vi "Find Straight Edge.vi"(6 "Analysis_Setting IN":T2={"PreProcess"=enum."*Algorithm*", "Parameter"=""}, 8 "error in (no error)":errorcluster, 9 "ProjectName":string, 10 "ROI List IN":refnum<vi>, 11 "Vision_Image":T12(plugin-control)) -> (0 "error out":errorcluster, 1 "Cancel?":bool, 3 "Analysis_Setting":T2={"PreProcess"=enum."*Algorithm*", "Parameter"=""})   [LabVIEW 2019]
uses:
  <vilib>/userdefined/High Color/IMAQdx.ctl
  <vilib>/vision/NI_Vision_Development_Module.lvlib
  Controls/Analysis_Type.ctl
  Controls/Analysis_Setting.ctl
  Controls/_UI Command Cluster/Find Straight Edge_UI Command Cluster.ctl
  Controls/Find Straight Edge/Analysis_Find Straight Edge_Parameter.ctl
  <vilib>/vision/Measure.llb/Straight Edge Process.ctl
  <vilib>/vision/Measure.llb/Straight Edge Options.ctl
  <vilib>/vision/Measure.llb/Edge Polarity.ctl
  <vilib>/vision/Measure.llb/Edge Options.ctl
  Controls/V_Analysis_Type.ctl
  Ctrl/VisionProcessName.ctl
panel:
  in  "Number of Matches Requested":i32=1 min=1 max=9999
  in  "Snap?":bool
  out "Edge Info Size":i32
  in  "ROI":T1
  out "Numeric":i32
  in  "Done":bool
  in  "Straight Edge_UI Command":T4(ring)
  in  "Cancel":bool
  in  "Straight EdgeTab":T5(tab)
  in  "Options":T8={"Search Direction"=0, "Edge Options"={"Edge Polarity"=0, "Kernel Size"=3, "Width"=3, "Minimum Edge Strength"=10.0, "Interpolation Type"=enum."Bilinear Fixed", "Data Processing Method"=enum."Average"}, "Show Search Area"=FALSE, "Show Search Lines"=FALSE, "Show Edges Found"=FALSE, "Show Result"=TRUE, "Search Area Color"=65280, "Search Lines Color"=255, "Edge Locations Color"=16776960, "Result Color"=16711680, "Overlay Group Name"=""} {"Edge Options"."Edge Polarity" items=["All Edges", "Rising Edges", "Falling Edges"]; "Edge Options"."Minimum Edge Strength" format="%.2f"; "Edge Options"."Width" step=2; "Edge Options"."Kernel Size" min=3 step=2; "Search Direction" items=["Left to Right", "Right to Left", "Top to Bottom", "Bottom to Top"]}
  in  "Line Fit Options":T9={"Number of Lines"=1, "Type"=enum."First Edge Rake", "Min. Score"=10.0, "Max. Score"=1000.0, "Orientation"=0.0, "Angle Range"=45.0, "Angle Tolerance"=1.0, "Step Size"=7, "Min. SNR (db)"=0.0, "Min. Points (%)"=25.0, "Hough Iterations"=5} {"Min. Points (%)" min=0.0 max=100.0; "Min. SNR (db)" min=0.0; "Max. Score" min=0.0 max=1024.0; "Min. Score" min=0.0 max=1024.0 step=1.0}
  out "Straight Edges":T11(array[cluster]) {"Point2 (Real-World)"."Y" format="%.2f"; "Point2 (Real-World)"."X" format="%.2f"; "Point1 (Real-World)"."Y" format="%.2f"; "Point1 (Real-World)"."X" format="%.2f"; "Point2 (Pixels)"."Y" format="%.2f"; "Point2 (Pixels)"."X" format="%.2f"; "Point1 (Pixels)"."Y" format="%.2f"; "Point1 (Pixels)"."X" format="%.2f"}
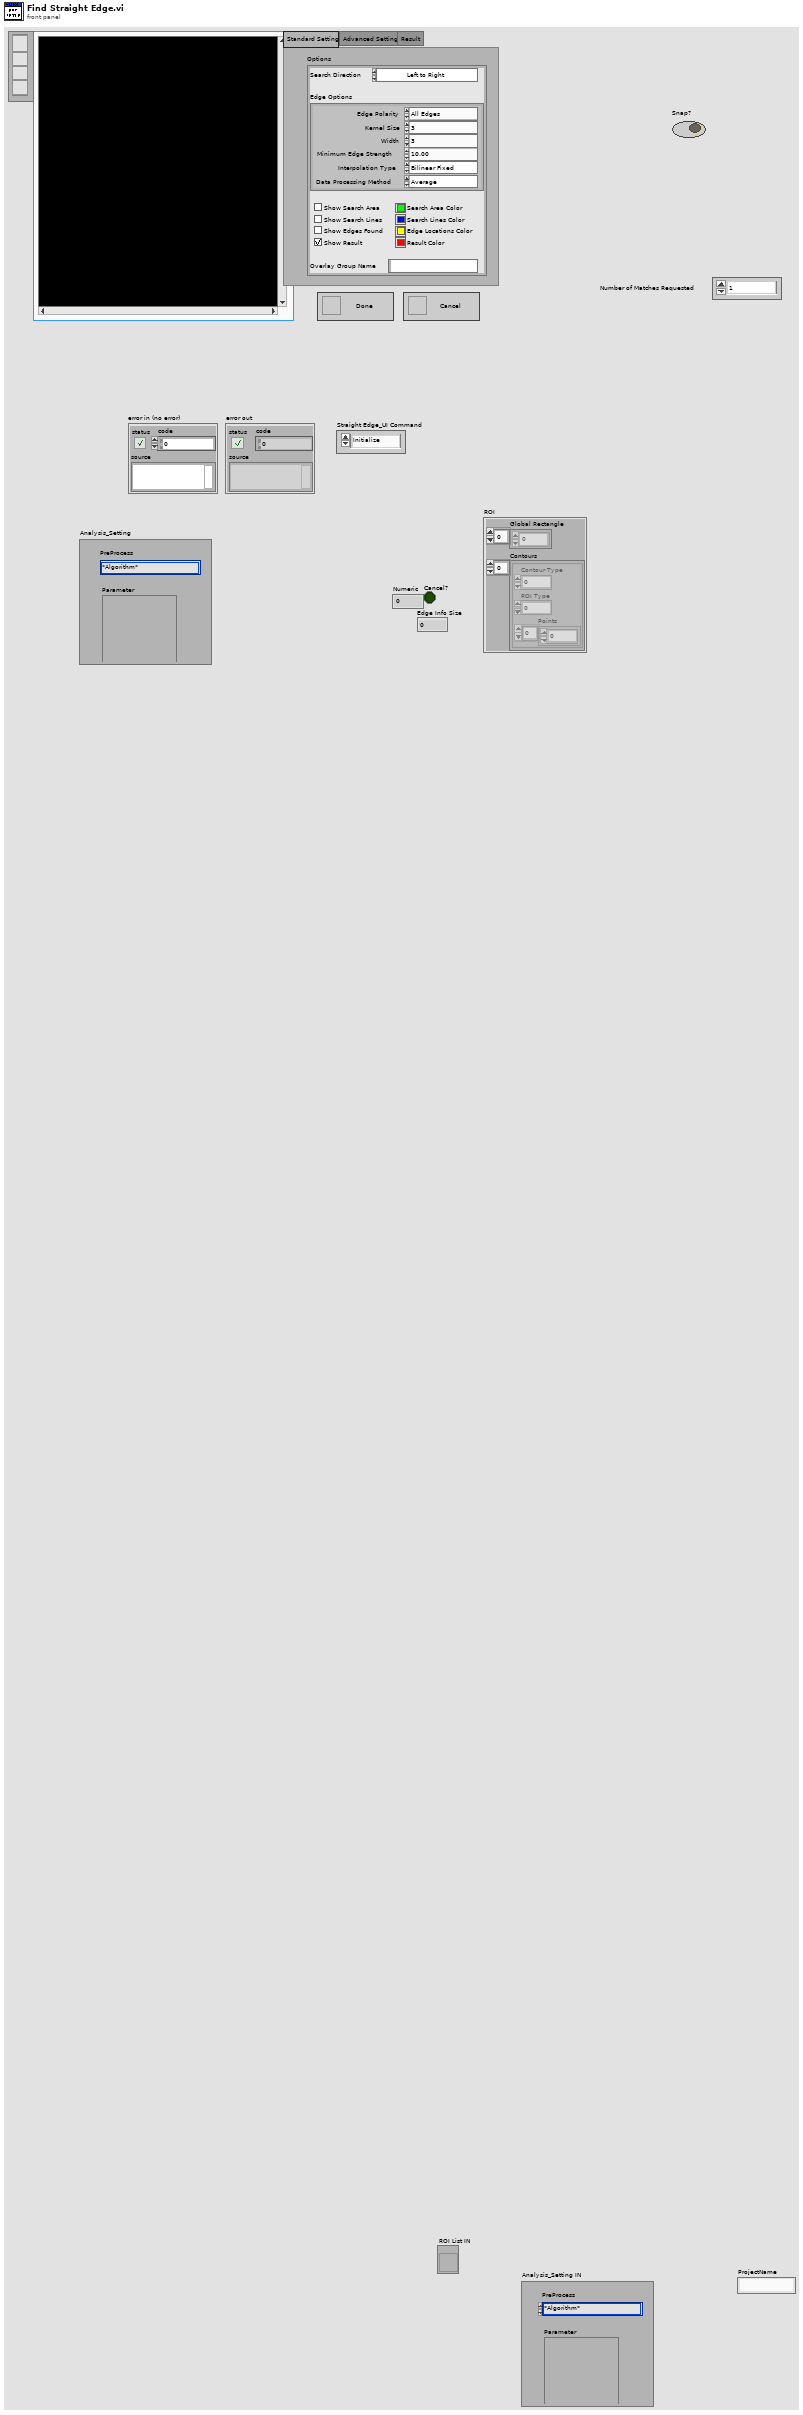
[diagram p1: front panel]
types:
  T1 = cluster{"Global Rectangle":i32[], "Contours":cluster{"Contour Type":u32, "ROI Type":u32, "Points":i32[]}[]}
  T2 = typedef "Analysis_Setting.ctl" = cluster{"PreProcess":T3, "Parameter":string}
  T3 = typedef "VisionProcessName.ctl" = enum16{"*CamParameter*", "CamAttributes", "*Preprocess*", "CG_Brightness", "C_Plane Extraction", "C_Threshold", "G_Lookup Table", "G_Threshold", "B_Image Inversion", "*Algorithm*", "CG_Histogram", "C_Color Matching", "C_Color Pattern Matching", "G_PatternMatch", "CG_Find Straight Edge", "CG_Adv. Find Straight Edge", "CG_Find Circular Edge", "G_Max Clamp", "G_Clamp (Rake)", "G_Pattern Matching"}
  T4 = enum16{"Initialize", "Done", "Run Algorithm", "Cancel"}
  T5 = enum32{"Standard Setting", "Advanced Setting", "Result"}
  T6 = typedef "Edge Options.ctl" = cluster{"Edge Polarity":T7, "Kernel Size":u32, "Width":u32, "Minimum Edge Strength":sgl, "Interpolation Type":enum32{"Zero Order", "Bilinear", "Quadratic", "Cubic", "Bilinear Fixed"}, "Data Processing Method":enum32{"Average", "Median"}}
  T7 = typedef "Edge Polarity.ctl" = u32
  T8 = cluster{"Search Direction":u32, "Edge Options":T6, "Show Search Area":bool, "Show Search Lines":bool, "Show Edges Found":bool, "Show Result":bool, "Search Area Color":u32, "Search Lines Color":u32, "Edge Locations Color":u32, "Result Color":u32, "Overlay Group Name":string}
  T9 = typedef "Straight Edge Options.ctl" = cluster{"Number of Lines":i32, "Type":T10, "Min. Score":dbl, "Max. Score":dbl, "Orientation":dbl, "Angle Range":dbl, "Angle Tolerance":dbl, "Step Size":u32, "Min. SNR (db)":dbl, "Min. Points (%)":dbl, "Hough Iterations":i32}
  T10 = typedef "Straight Edge Process.ctl" = enum32{"First Edge Rake", "Best Edge Rake", "Hough Edge Rake", "First Edge Projection", "Best Edge Projection"}
  T11 = cluster{"Point1 (Pixels)":cluster{"X":sgl, "Y":sgl}, "Point2 (Pixels)":cluster{"X":sgl, "Y":sgl}, "Point1 (Real-World)":cluster{"X":sgl, "Y":sgl}, "Point2 (Real-World)":cluster{"X":sgl, "Y":sgl}, "Angle (Pixel)":dbl, "Angle (Real-World)":dbl, "Score":dbl, "Straightness":dbl, "Average SNR (db)":dbl, "Calibration Valid":bool}[]
  T12 = typedef "IMAQ Image.ctl" = refnum<image>
  T13 = typedef "Find Straight Edge_UI Command Cluster.ctl" = cluster{"Find Straight Edge_UI Command":enum16{"Initialize", "Done", "Run Algorithm", "Cancel"}, "Snap Simulation Mouse Down":bool, "ROI Descriptor":cluster{"Global Rectangle":i32[], "Contours":cluster{"Contour Type":u32, "ROI Type":u32, "Points":i32[]}[]}, "Number of Matches Requested":i32, "Options":cluster{"Search Direction":u32, "Edge Options":T6, "Show Search Area":bool, "Show Search Lines":bool, "Show Edges Found":bool, "Show Result":bool, "Search Area Color":u32, "Search Lines Color":u32, "Edge Locations Color":u32, "Result Color":u32, "Overlay Group Name":string}, "Line Fit Options":T9}
  T14 = typedef "IMAQ Line" = cluster{"Start X":i32, "Start Y":i32, "End X":i32, "End Y":i32}
  T15 = typedef "IMAQdx.ctl" = refnum<k21>
  T16 = cluster{"Contour Type":u32, "ROI Type":u32, "Points":i32[]}
  T17 = typedef "Image Type" = u32
  T18 = typedef "Analysis_Find Straight Edge_Parameter.ctl" = cluster{"ROI Descriptor":cluster{"Global Rectangle":i32[], "Contours":cluster{"Contour Type":u32, "ROI Type":u32, "Points":i32[]}[]}, "Number of Matches Requested":i32, "Edge Info Size":i32, "Options":cluster{"Search Direction":u32, "Edge Options":T6, "Show Search Area":bool, "Show Search Lines":bool, "Show Edges Found":bool, "Show Result":bool, "Search Area Color":u32, "Search Lines Color":u32, "Edge Locations Color":u32, "Result Color":u32, "Overlay Group Name":string}, "Line Fit Options":T9}
  T19 = typedef "Analysis_Type.ctl" = u16
  T20 = typedef "Analysis_Setting.ctl" = cluster{"PreProcess":T21, "Parameter":string}
  T21 = typedef "V_Analysis_Type.ctl" = enum16{"None", "C_Color Pattern Matching", "G_PatternMatching", "G_ShapeDectect", "G_GeometricMatch", "B_Area Check"}
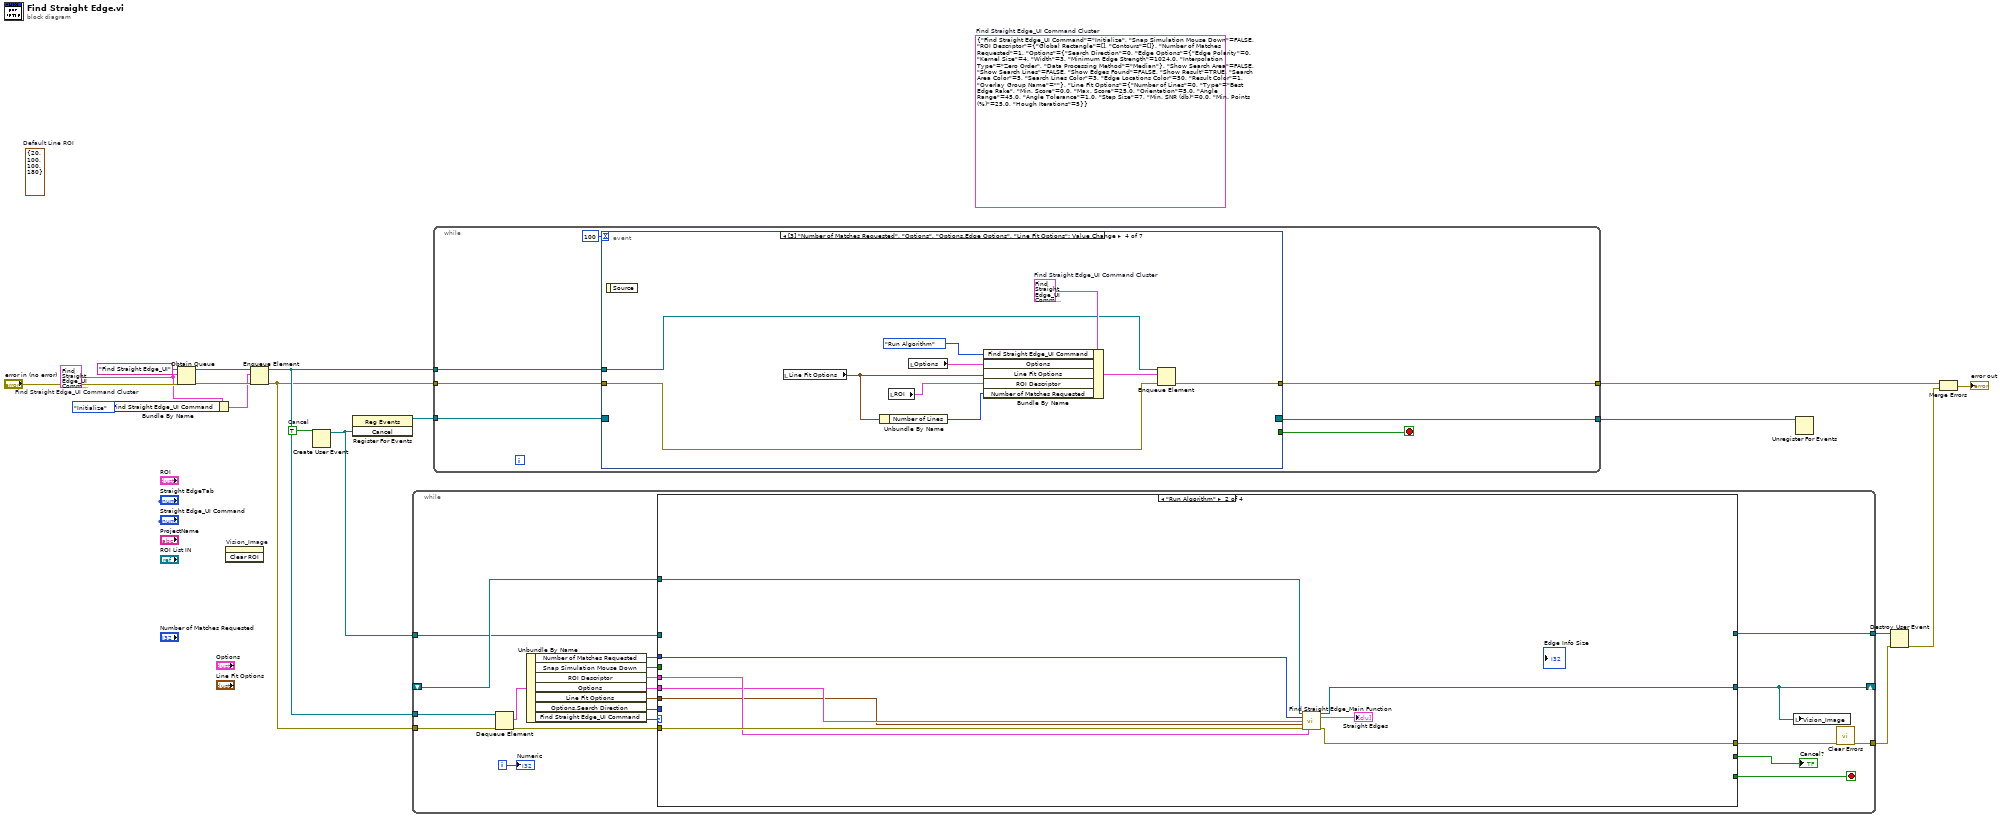
[diagram p0: block diagram]
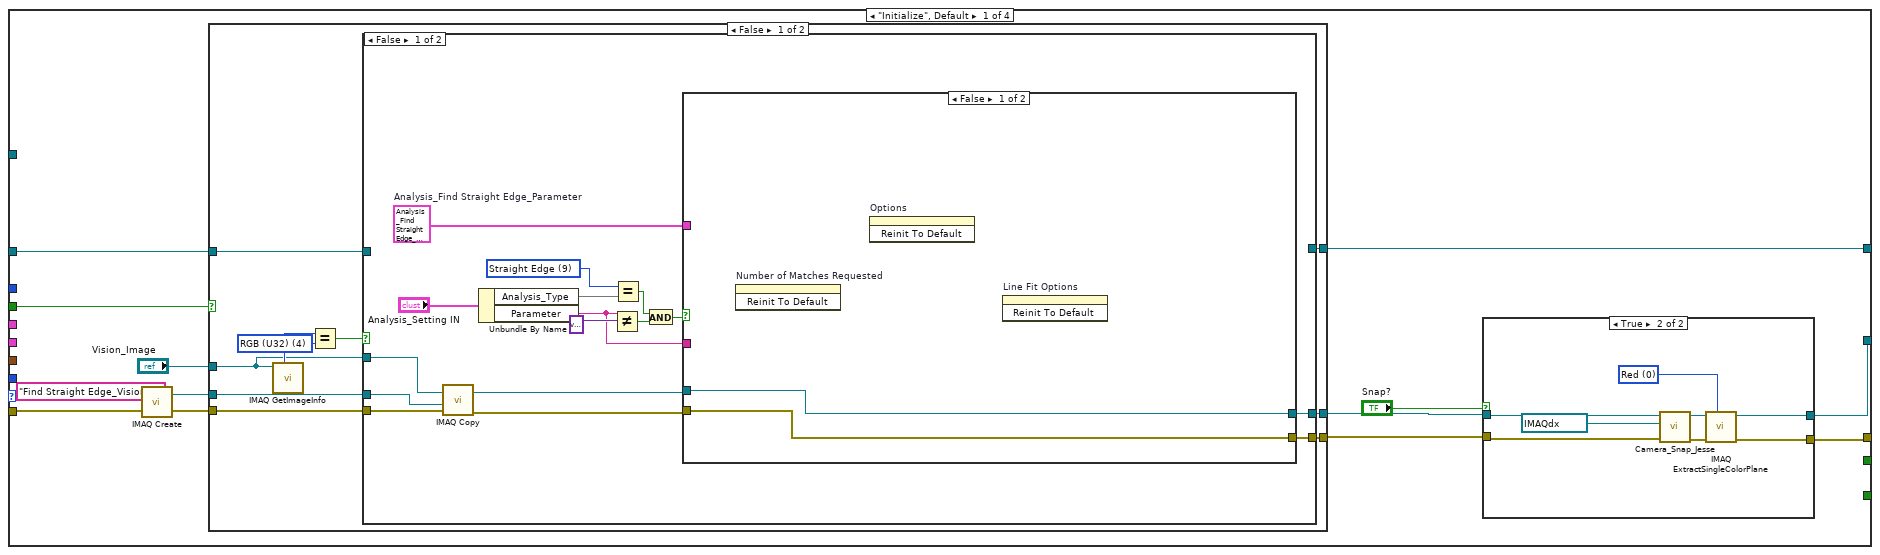
[diagram p2: hidden frame]
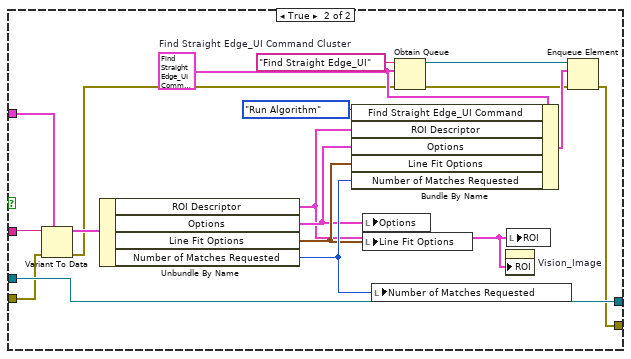
[diagram p4: hidden frame]
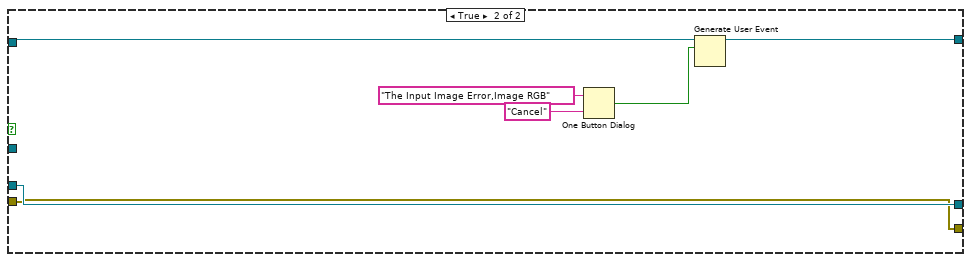
[diagram p5: hidden frame]
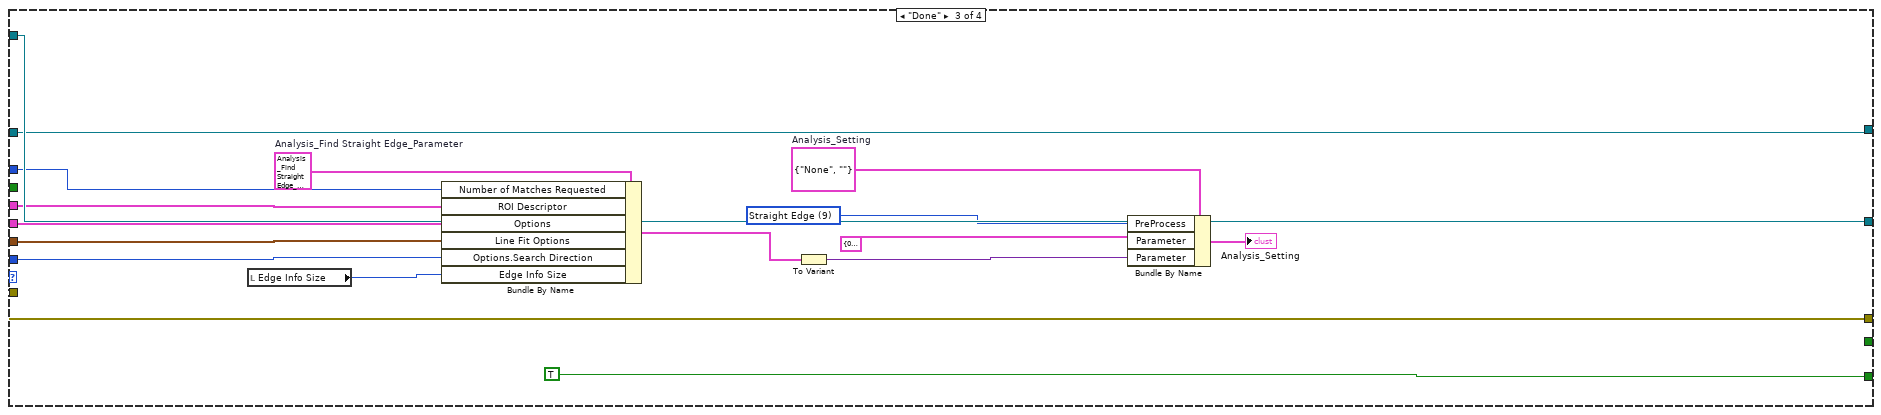
[diagram p7: hidden frame]
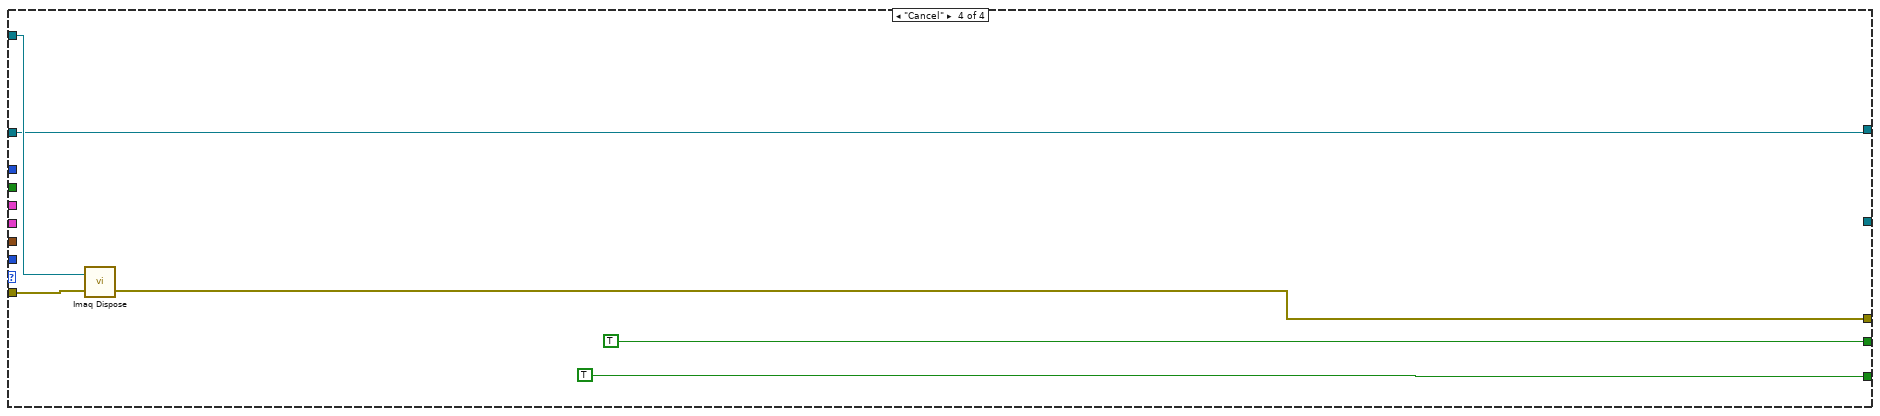
[diagram p8: hidden frame]
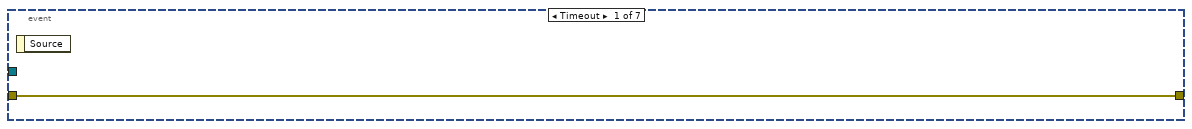
[diagram p9: hidden frame]
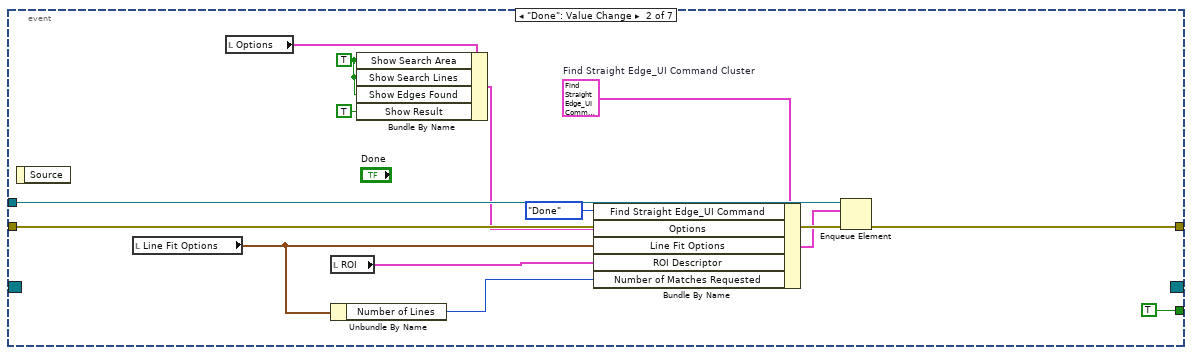
[diagram p10: hidden frame]
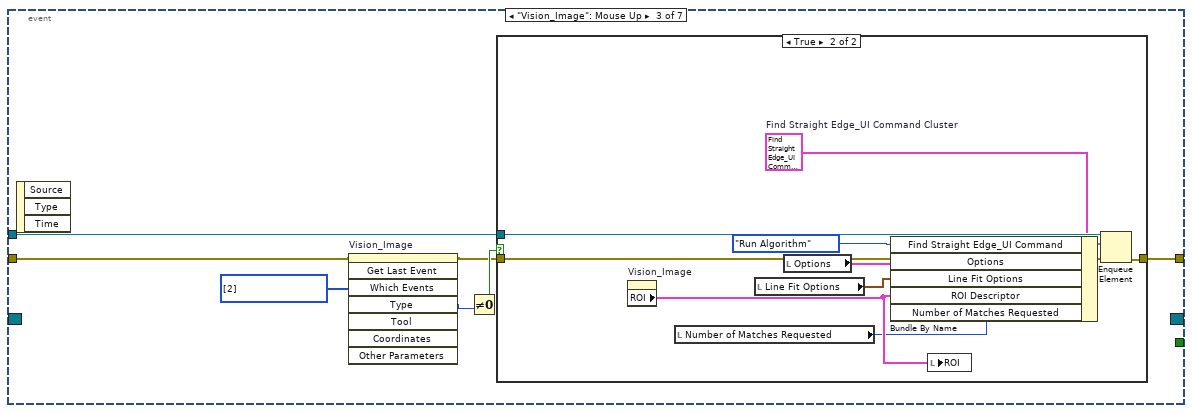
[diagram p11: hidden frame]
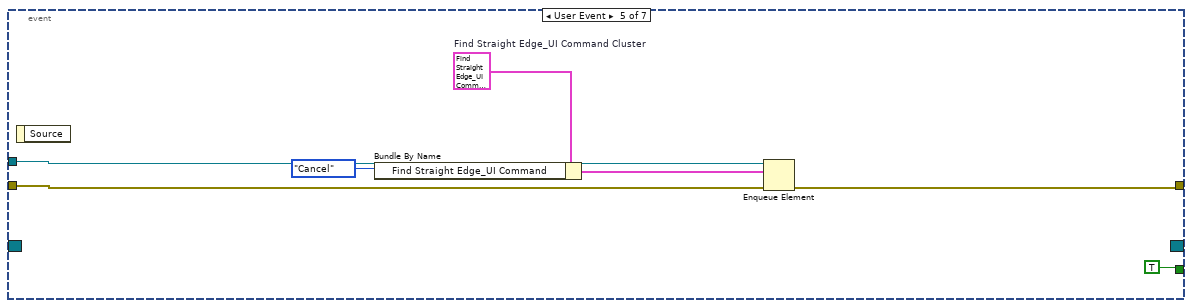
[diagram p13: hidden frame]
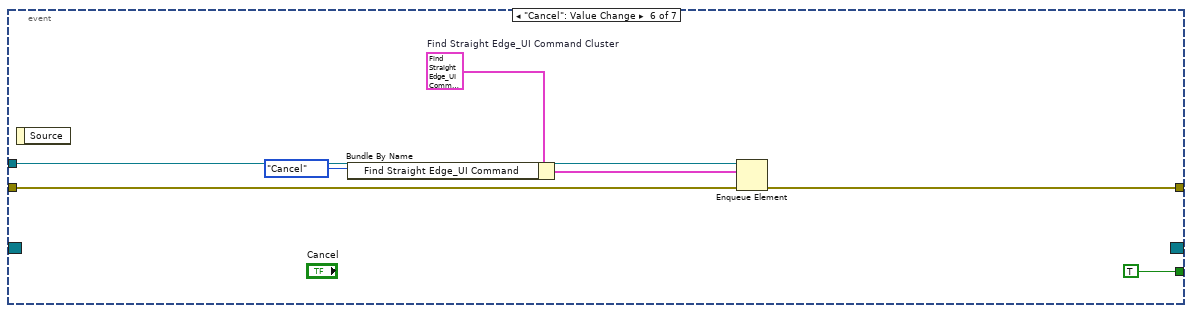
[diagram p14: hidden frame]
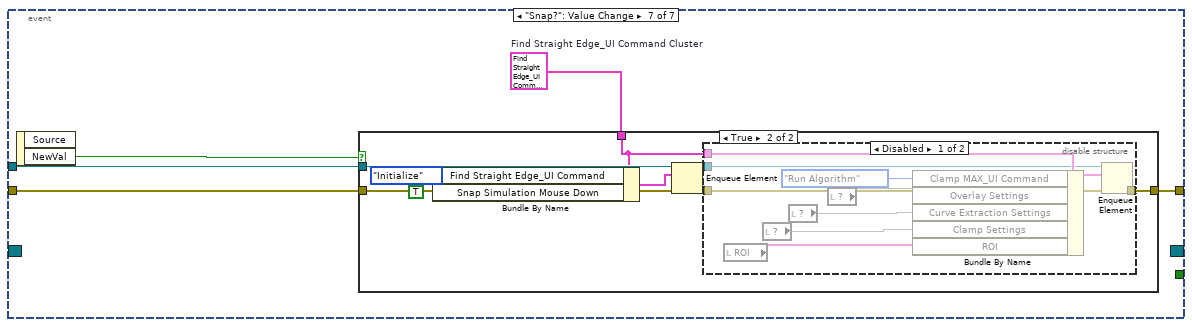
[diagram p15: hidden frame]
diagram:
  (unwired) T13 {"Find Straight Edge_UI Command"=enum."Initialize", "Snap Simulation Mouse Down"=FALSE, "ROI Descriptor"={"Global Rectangle"=[], "Contours"=[]}, "Number of Matches Requested"=1, "Options"={"Search Direction"=0, "Edge Options"={"Edge Polarity"=0, "Kernel Size"=4, "Width"=3, "Minimum Edge Strength"=1024.0, "Interpolation Type"=enum."Zero Order", "Data Processing Method"=enum."Median"}, "Show Search Area"=FALSE, "Show Search Lines"=FALSE, "Show Edges Found"=FALSE, "Show Result"=TRUE, "Search Area Color"=5, "Search Lines Color"=3, "Edge Locations Color"=50, "Result Color"=1, "Overlay Group Name"=""}, "Line Fit Options"={"Number of Lines"=0, "Type"=enum."Best Edge Rake", "Min. Score"=0.0, "Max. Score"=25.0, "Orientation"=5.0, "Angle Range"=45.0, "Angle Tolerance"=1.0, "Step Size"=7, "Min. SNR (db)"=0.0, "Min. Points (%)"=25.0, "Hough Iterations"=5}}  # Find Straight Edge_UI Command Cluster
  w7 = TRUE  # Cancel
  w8 = T13 {"Find Straight Edge_UI Command"=enum."Initialize", "Snap Simulation Mouse Down"=FALSE, "ROI Descriptor"={"Global Rectangle"=[], "Contours"=[]}, "Number of Matches Requested"=1, "Options"={"Search Direction"=0, "Edge Options"={"Edge Polarity"=0, "Kernel Size"=4, "Width"=3, "Minimum Edge Strength"=1024.0, "Interpolation Type"=enum."Zero Order", "Data Processing Method"=enum."Median"}, "Show Search Area"=FALSE, "Show Search Lines"=FALSE, "Show Edges Found"=FALSE, "Show Result"=TRUE, "Search Area Color"=5, "Search Lines Color"=3, "Edge Locations Color"=50, "Result Color"=1, "Overlay Group Name"=""}, "Line Fit Options"={"Number of Lines"=0, "Type"=enum."Best Edge Rake", "Min. Score"=0.0, "Max. Score"=25.0, "Orientation"=5.0, "Angle Range"=45.0, "Angle Tolerance"=1.0, "Step Size"=7, "Min. SNR (db)"=0.0, "Min. Points (%)"=25.0, "Hough Iterations"=5}}  # Find Straight Edge_UI Command Cluster
  (unwired) T14 {"Start X"=20, "Start Y"=100, "End X"=100, "End Y"=180}  # Default Line ROI
  n1 = Bundle By Name(cluster=w8, "Find Straight Edge_UI Command"=T4."Initialize" ("Barcode 1D_UI Command")) -> (w13:T13)
  n2 = Obtain Queue(name (unnamed)="Find Straight Edge_UI", element data type=w8, error in (no error)="error in (no error)") -> (queue out=w18:refnum<queue>, error out=w17:errorcluster)  [unwired: 2 in, 1 out]
  n3 = invoke on="Vision_Image" class="ImageControl" method="Clear ROI"() -> ()  [unwired: 3 in, 3 out]
  n4 = Enqueue Element(queue=w18, element=w13, error in (no error)=w17) -> (queue out=w12:refnum<queue>, error out=w11:errorcluster)  [unwired: 1 in, 1 out]
  n5 = Create User Event(user event datatype=w7) -> (user event=w4:refnum<user-event>)  [unwired: 1 in, 1 out]
  n6 = register-events(w4) -> (reference out=w6:refnum<event-registration>)  [unwired: 2 in, 1 out]
  n7 = while {
    tunnel: w12 -> [w38]
    tunnel: w11 -> [w37]
    shift-right: [w32] -> _
    shift-left: _ -> [w34]
    tunnel: [w20] -> w2
    tunnel: w4 -> [w22]
    tunnel: [w21] -> w3
    i -> [w33]
    stop <- w25 stop-if-true
    n8 = Dequeue Element(queue=w38, error in (no error)=w37) -> (element=w35:T13, error out=w36:errorcluster)  [unwired: 1 in, 2 out]
    n9 = Unbundle By Name(w35) -> ("Number of Matches Requested"=w23:i32, "Snap Simulation Mouse Down"=w27:bool, "ROI Descriptor"=w26:T1, "Options"=w30:T8, "Line Fit Options"=w29:T9, "Options.Search Direction"=w28:u32, "Find Straight Edge_UI Command"=w24:T4)
    n10 = case shown="\"Run Algorithm\"" w24 {
      tunnel: w36 -> [w50 w124 w139 w145]
      tunnel: [w41 w123 w139 w144] -> w19
      tunnel: [_ _ TRUE TRUE] -> w25
      tunnel: [w42 w122 w140 _] -> w32
      tunnel: w34 -> [_ w117 w140 w146]
      tunnel: [_ _ _ TRUE] -> w31
      tunnel: w30 -> [_ w119 w126 _]
      tunnel: w29 -> [_ w118 w127 _]
      tunnel: w28 -> [_ _ w130 _]
      tunnel: w27 -> [w49 _ _ _]
      tunnel: w26 -> [_ w121 w131 _]
      tunnel: w23 -> [_ w116 w129 _]
      tunnel: w22 -> [w40 _ w125 w142]
      tunnel: [w39 _ w125 w142] -> w21
      frame "Initialize", Default {
        n11 = call "IMAQ Create"("Image Name"="Find Straight Edge_Vision", "error in (no error)"=w50) -> ("New Image"=w47:T12, "error out"=w48:errorcluster)  [unwired: 3 in]
        n12 = case shown="False" w49 {
          tunnel: [w71 w115] -> w44
          tunnel: [w70 w114] -> w43
          tunnel: w48 -> [w69 w115]
          tunnel: w47 -> [w68 w114]
          tunnel: "Vision_Image" -> [w62 _]
          tunnel: w40 -> [w64 _]
          tunnel: [w63 _] -> w39
          frame False {
            w66 = T17 4 items=["Grayscale (U8)", "Grayscale (I16)", "Grayscale (SGL)", "Complex (CSG)", "RGB (U32)", "HSL (U32)", "RGB (U64)", "Grayscale (U16)"] ("y")
            n13 = call "IMAQ GetImageInfo"("Image"=w62) -> ("Image Type"=w67:T17)  [unwired: 3 in, 7 out]
            n14 = Equal?(x=w67, y=w66) -> (x = y?=w65:bool)
            n15 = case shown="False" w65 {
              tunnel: [w87 w112] -> w71
              tunnel: [w86 w113] -> w70
              tunnel: w69 -> [w77 w112]
              tunnel: w68 -> [w76 w113]
              tunnel: w64 -> [_ w108]
              tunnel: [_ w107] -> w63
              tunnel: w62 -> [w72 _]
              frame False {
                w73 = T18 {"ROI Descriptor"={"Global Rectangle"=[], "Contours"=[]}, "Number of Matches Requested"=1, "Edge Info Size"=0, "Options"={"Search Direction"=0, "Edge Options"={"Edge Polarity"=0, "Kernel Size"=4, "Width"=3, "Minimum Edge Strength"=1024.0, "Interpolation Type"=enum."Zero Order", "Data Processing Method"=enum."Median"}, "Show Search Area"=FALSE, "Show Search Lines"=FALSE, "Show Edges Found"=FALSE, "Show Result"=TRUE, "Search Area Color"=5, "Search Lines Color"=3, "Edge Locations Color"=50, "Result Color"=1, "Overlay Group Name"=""}, "Line Fit Options"={"Number of Lines"=0, "Type"=enum."Best Edge Rake", "Min. Score"=0.0, "Max. Score"=25.0, "Orientation"=5.0, "Angle Range"=45.0, "Angle Tolerance"=1.0, "Step Size"=7, "Min. SNR (db)"=0.0, "Min. Points (%)"=25.0, "Hough Iterations"=5}}  # Analysis_Find Straight Edge_Parameter
                w83 = T19 9 items=["None", "PatternMatch", "Edge Detection", "Barcode 1D", "Barcode 2D", "Clamp", "Clamp MAX", "Particle", "Histogram", "Straight Edge", "Circle", "Shape Detect", "OCR", "Contour", "ColorMatch"] ("x")
                n16 = call "IMAQ Copy"("error in (no error)"=w77, "Image Dst"=w76, "Image Src"=w72) -> ("error out"=w75:errorcluster, "Image Dst Out"=w74:T12)  [unwired: 3 in]
                n17 = Unbundle By Name("Analysis_Setting IN") -> ("Analysis_Type"=w82, "Parameter"=w78:string)
                n18 = Not Equal?(x=w78, y=variant) -> (x != y?=w84:bool)
                n19 = Equal?(x=w83, y=w82) -> (x = y?=w85:bool)
                n20 = And(x=w85, y=w84) -> (x .and. y?=w79:bool)
                n21 = case shown="False" w79 {
                  tunnel: [w88 w94] -> w87
                  tunnel: [w89 w106] -> w86
                  tunnel: w75 -> [w88 w96]
                  tunnel: w74 -> [w89 w106]
                  tunnel: w78 -> [_ w105]
                  tunnel: w73 -> [_ w97]
                  frame False {
                    n22 = invoke on="Number of Matches Requested" class="DigNum (strict)" method="Reinit To Default"() -> ()  [unwired: 3 in, 3 out]
                    n23 = invoke on="Options" class="Clust (strict)" method="Reinit To Default"() -> ()  [unwired: 3 in, 3 out]
                    n24 = invoke on="Line Fit Options" class="Clust (strict)" method="Reinit To Default"() -> ()  [unwired: 3 in, 3 out]
                  }
                  frame True {
                    w103 = T13 {"Find Straight Edge_UI Command"=enum."Initialize", "Snap Simulation Mouse Down"=FALSE, "ROI Descriptor"={"Global Rectangle"=[], "Contours"=[]}, "Number of Matches Requested"=1, "Options"={"Search Direction"=0, "Edge Options"={"Edge Polarity"=0, "Kernel Size"=4, "Width"=3, "Minimum Edge Strength"=1024.0, "Interpolation Type"=enum."Zero Order", "Data Processing Method"=enum."Median"}, "Show Search Area"=FALSE, "Show Search Lines"=FALSE, "Show Edges Found"=FALSE, "Show Result"=TRUE, "Search Area Color"=5, "Search Lines Color"=3, "Edge Locations Color"=50, "Result Color"=1, "Overlay Group Name"=""}, "Line Fit Options"={"Number of Lines"=0, "Type"=enum."Best Edge Rake", "Min. Score"=0.0, "Max. Score"=25.0, "Orientation"=5.0, "Angle Range"=45.0, "Angle Tolerance"=1.0, "Step Size"=7, "Min. SNR (db)"=0.0, "Min. Points (%)"=25.0, "Hough Iterations"=5}}  # Find Straight Edge_UI Command Cluster
                    n25 = Variant To Data(error in=w96, type=w97, Variant=w105) -> (data=w104:T18, error out=w95:errorcluster)
                    n26 = Unbundle By Name(w104) -> ("ROI Descriptor"=w90:T1, "Options"=w91:T8, "Line Fit Options"=w92:T9, "Number of Matches Requested"=w93:i32)
                    n27 = Bundle By Name(cluster=w103, "Find Straight Edge_UI Command"=T4."Run Algorithm" ("Barcode 1D_UI Command"), "ROI Descriptor"=w90, "Options"=w91, "Line Fit Options"=w92, "Number of Matches Requested"=w93) -> (w102:T13)
                    n28 = local write "Options"(w91) -> ()
                    n29 = local write "Line Fit Options"(w92) -> ()
                    n30 = local write "Number of Matches Requested"(w93) -> ()
                    n31 = Obtain Queue(name (unnamed)="Find Straight Edge_UI", element data type=w103, error in (no error)=w95) -> (queue out=w98:refnum<queue>, error out=w99:errorcluster)  [unwired: 2 in, 1 out]
                    n32 = property on="Vision_Image" class="ImageControl"("ROI"=w90) -> ()  [unwired: 2 in, 2 out]
                    n33 = local write "ROI"(w90) -> ()
                    n34 = Enqueue Element(queue=w98, element=w102, error in (no error)=w99) -> (error out=w94:errorcluster)  [unwired: 1 in, 2 out]
                  }
                }
              }
              frame True {
                n35 = One Button Dialog(message="The Input Image Error,Image RGB", button name ("OK")="Cancel") -> (true=w109:bool)
                n36 = Generate User Event(user event=w108, event data cluster=w109) -> (user event out=w107:refnum<user-event>)  [unwired: 2 in, 1 out]
              }
            }
          }
          frame True {
          }
        }
        n37 = case shown="True" "Snap?" {
          tunnel: [w52 w57] -> w41
          tunnel: [w53 w56] -> w42
          tunnel: w44 -> [w52 w54]
          tunnel: w43 -> [w53 w55]
          frame False {
          }
          frame True {
            w59 = 0 items=["Red", "Green", "Blue", "Hue", "Saturation", "Luminance", "Value", "Intensity"] ("Color Plane")
            n38 = call "Camera_Snap_Jesse.vi"("error in (no error)"=w54, "Camera Session In"=T15 "cam01", "Image In"=w55) -> ("error out"=w58:errorcluster, "New Image"=w60:T12)  [unwired: 7 in]
            n39 = call "IMAQ ExtractSingleColorPlane"("Color Plane"=w59, "error in (no error)"=w58, "Image Src"=w60) -> ("error out"=w57:errorcluster, "Image Dst Out"=w56:T12)  [unwired: 1 in, 6 out]
          }
        }
      }
      frame "Run Algorithm" {
        n40 = call "Find Straight Edge_Main Function.vi"("Refnum in"=w117, "Number of Matches Requested"=w116, "Options"=w119, "Line Fit Options"=w118, "error in (no error)"=w124, "ROI"=w121) -> ("Refnum out"=w122:T12, "Straight Edges"=→"Straight Edges":T11, "error out"=w123:errorcluster)  [unwired: 7 in]
      }
      frame "Done" {
        w132 = T18 {"ROI Descriptor"={"Global Rectangle"=[], "Contours"=[]}, "Number of Matches Requested"=1, "Edge Info Size"=0, "Options"={"Search Direction"=0, "Edge Options"={"Edge Polarity"=0, "Kernel Size"=4, "Width"=3, "Minimum Edge Strength"=1024.0, "Interpolation Type"=enum."Zero Order", "Data Processing Method"=enum."Median"}, "Show Search Area"=FALSE, "Show Search Lines"=FALSE, "Show Edges Found"=FALSE, "Show Result"=TRUE, "Search Area Color"=5, "Search Lines Color"=3, "Edge Locations Color"=50, "Result Color"=1, "Overlay Group Name"=""}, "Line Fit Options"={"Number of Lines"=0, "Type"=enum."Best Edge Rake", "Min. Score"=0.0, "Max. Score"=25.0, "Orientation"=5.0, "Angle Range"=45.0, "Angle Tolerance"=1.0, "Step Size"=7, "Min. SNR (db)"=0.0, "Min. Points (%)"=25.0, "Hough Iterations"=5}}  # Analysis_Find Straight Edge_Parameter
        w133 = T19 9 items=["None", "PatternMatch", "Edge Detection", "Barcode 1D", "Barcode 2D", "Clamp", "Clamp MAX", "Particle", "Histogram", "Straight Edge", "Circle", "Shape Detect", "OCR", "Contour", "ColorMatch"] ("Analysis_Type")
        w138 = T20 {"PreProcess"=enum."None", "Parameter"=""}  # Analysis_Setting
        n41 = local read "Edge Info Size"() -> (w128:i32)
        n42 = Bundle By Name(cluster=w132, "Number of Matches Requested"=w129, "ROI Descriptor"=w131, "Options"=w126, "Line Fit Options"=w127, "Options.Search Direction"=w130, "Edge Info Size"=w128) -> (w136:T18)
        n43 = To Variant(anything=w136) -> (Variant=w135:variant)
        n44 = Bundle By Name(cluster=w138, "PreProcess"=w133, "Parameter"=T16 {"Contour Type"=0, "ROI Type"=0, "Points"=[]} ("RegionContour"), "Parameter"=w135) -> (→"Analysis_Setting":T20)
      }
      frame "Cancel" {
        n45 = call "Imaq Dispose"("Image"=w146, "error in (no error)"=w145) -> ("error out"=w144:errorcluster)  [unwired: 4 in]
      }
    }
    "Cancel?" <- w31
    n46 = local write "Vision_Image"(w32) -> ()
    n47 = call <vilib>:"Clear Errors.vi"("error in (no error)"=w19) -> ("error out"=w20:errorcluster)  [unwired: 5 in, 1 out]
    "Numeric" <- w33
  }
  n48 = while {
    tunnel: w12 -> [w154]
    tunnel: w11 -> [w153]
    tunnel: [w152] -> w15
    tunnel: w6 -> [w149]
    tunnel: [w148] -> w5
    stop <- w150 stop-if-true
    n49 = event shown="[3] \"Number of Matches Requested\", \"Options\", \"Options.Edge Options\", \"Line Fit Options\": Value Change" {
      selector: w149 -> [_ _ _ _ _ _ _]
      dyn-events: [_ _ _ _ _ _ _] -> w148
      timeout: 100 -> [_ _ _ _ _ _ _]
      tunnel: w154 -> [_ w169 w176 w191 w200 w211 w216]
      tunnel: w153 -> [w155 w168 w173 w190 w199 w210 w215]
      tunnel: [_ TRUE _ _ TRUE TRUE _] -> w150
      tunnel: [w155 w167 w170 w197 w198 w208 w214] -> w152
      event Timeout {
        n50 = event-data() -> ()  [unwired: 1 in, 1 out]
      }
      event "Done": Value Change {
        w158 = TRUE ("Show Search Area")
        w166 = T13 {"Find Straight Edge_UI Command"=enum."Initialize", "Snap Simulation Mouse Down"=FALSE, "ROI Descriptor"={"Global Rectangle"=[], "Contours"=[]}, "Number of Matches Requested"=1, "Options"={"Search Direction"=0, "Edge Options"={"Edge Polarity"=0, "Kernel Size"=4, "Width"=3, "Minimum Edge Strength"=1024.0, "Interpolation Type"=enum."Zero Order", "Data Processing Method"=enum."Median"}, "Show Search Area"=FALSE, "Show Search Lines"=FALSE, "Show Edges Found"=FALSE, "Show Result"=TRUE, "Search Area Color"=5, "Search Lines Color"=3, "Edge Locations Color"=50, "Result Color"=1, "Overlay Group Name"=""}, "Line Fit Options"={"Number of Lines"=0, "Type"=enum."Best Edge Rake", "Min. Score"=0.0, "Max. Score"=25.0, "Orientation"=5.0, "Angle Range"=45.0, "Angle Tolerance"=1.0, "Step Size"=7, "Min. SNR (db)"=0.0, "Min. Points (%)"=25.0, "Hough Iterations"=5}}  # Find Straight Edge_UI Command Cluster
        n51 = event-data() -> ()  [unwired: 1 in, 1 out]
        n52 = local read "Line Fit Options"() -> (w157:T9)
        n53 = local read "Options"() -> (w161:T8)
        n54 = local read "ROI"() -> (w162:T1)
        n55 = Unbundle By Name(w157) -> ("Number of Lines"=w156:i32)
        n56 = Bundle By Name(cluster=w161, "Show Search Area"=w158, "Show Search Lines"=w158, "Show Edges Found"=w158, "Show Result"=TRUE) -> (w160:T8)
        n57 = Bundle By Name(cluster=w166, "Find Straight Edge_UI Command"=T4."Done" ("Edge Detection_UI Command"), "Options"=w160, "Line Fit Options"=w157, "ROI Descriptor"=w162, "Number of Matches Requested"=w156) -> (w164:T13)
        n58 = Enqueue Element(queue=w169, element=w164, error in (no error)=w168) -> (error out=w167:errorcluster)  [unwired: 1 in, 2 out]
      }
      event "Vision_Image": Mouse Up {
        w174 = i32[] [2] items=["No Event"=0, "Click Event"=1, "Draw Event"=2, "Size Event"=4, "Scroll Event"=5, "Double Click Event"=8] ("Which Events")
        n59 = event-data() -> ()  [unwired: 1 in, 3 out]
        n60 = invoke on="Vision_Image" class="ImageControl" method="Get Last Event"(error in=w173, "Which Events"=w174) -> (error out=w172:errorcluster, "Type"=w171:i32)  [unwired: 6 in, 6 out]
        n61 = Not Equal To 0?(x=w171) -> (x != 0?=w175:bool)
        n62 = case shown="True" w175 {
          tunnel: w176 -> [_ w185]
          tunnel: w172 -> [w177 w187]
          tunnel: [w177 w186] -> w170
          frame False {
          }
          frame True {
            w184 = T13 {"Find Straight Edge_UI Command"=enum."Initialize", "Snap Simulation Mouse Down"=FALSE, "ROI Descriptor"={"Global Rectangle"=[], "Contours"=[]}, "Number of Matches Requested"=1, "Options"={"Search Direction"=0, "Edge Options"={"Edge Polarity"=0, "Kernel Size"=4, "Width"=3, "Minimum Edge Strength"=1024.0, "Interpolation Type"=enum."Zero Order", "Data Processing Method"=enum."Median"}, "Show Search Area"=FALSE, "Show Search Lines"=FALSE, "Show Edges Found"=FALSE, "Show Result"=TRUE, "Search Area Color"=5, "Search Lines Color"=3, "Edge Locations Color"=50, "Result Color"=1, "Overlay Group Name"=""}, "Line Fit Options"={"Number of Lines"=0, "Type"=enum."Best Edge Rake", "Min. Score"=0.0, "Max. Score"=25.0, "Orientation"=5.0, "Angle Range"=45.0, "Angle Tolerance"=1.0, "Step Size"=7, "Min. SNR (db)"=0.0, "Min. Points (%)"=25.0, "Hough Iterations"=5}}  # Find Straight Edge_UI Command Cluster
            n63 = property on="Vision_Image" class="ImageControl"() -> ("ROI"=w181:T1)  [unwired: 2 in, 2 out]
            n64 = local read "Number of Matches Requested"() -> (w180:i32)
            n65 = local read "Line Fit Options"() -> (w178:T9)
            n66 = local read "Options"() -> (w179:T8)
            n67 = Bundle By Name(cluster=w184, "Find Straight Edge_UI Command"=T4."Run Algorithm" ("Clamp MAX_UI Command"), "Options"=w179, "Line Fit Options"=w178, "ROI Descriptor"=w181, "Number of Matches Requested"=w180) -> (w183:T13)
            n68 = local write "ROI"(w181) -> ()
            n69 = Enqueue Element(queue=w185, element=w183, error in (no error)=w187) -> (error out=w186:errorcluster)  [unwired: 1 in, 2 out]
          }
        }
      }
      event "Number of Matches Requested", "Options": Value Change {
        w196 = T13 {"Find Straight Edge_UI Command"=enum."Initialize", "Snap Simulation Mouse Down"=FALSE, "ROI Descriptor"={"Global Rectangle"=[], "Contours"=[]}, "Number of Matches Requested"=1, "Options"={"Search Direction"=0, "Edge Options"={"Edge Polarity"=0, "Kernel Size"=4, "Width"=3, "Minimum Edge Strength"=1024.0, "Interpolation Type"=enum."Zero Order", "Data Processing Method"=enum."Median"}, "Show Search Area"=FALSE, "Show Search Lines"=FALSE, "Show Edges Found"=FALSE, "Show Result"=TRUE, "Search Area Color"=5, "Search Lines Color"=3, "Edge Locations Color"=50, "Result Color"=1, "Overlay Group Name"=""}, "Line Fit Options"={"Number of Lines"=0, "Type"=enum."Best Edge Rake", "Min. Score"=0.0, "Max. Score"=25.0, "Orientation"=5.0, "Angle Range"=45.0, "Angle Tolerance"=1.0, "Step Size"=7, "Min. SNR (db)"=0.0, "Min. Points (%)"=25.0, "Hough Iterations"=5}}  # Find Straight Edge_UI Command Cluster
        n70 = event-data() -> ()  [unwired: 1 in, 1 out]
        n71 = local read "Line Fit Options"() -> (w189:T9)
        n72 = Unbundle By Name(w189) -> ("Number of Lines"=w188:i32)
        n73 = local read "ROI"() -> (w193:T1)
        n74 = local read "Options"() -> (w192:T8)
        n75 = Bundle By Name(cluster=w196, "Find Straight Edge_UI Command"=T4."Run Algorithm" ("Barcode 1D_UI Command"), "Options"=w192, "Line Fit Options"=w189, "ROI Descriptor"=w193, "Number of Matches Requested"=w188) -> (w194:T13)
        n76 = Enqueue Element(queue=w191, element=w194, error in (no error)=w190) -> (error out=w197:errorcluster)  [unwired: 1 in, 2 out]
      }
      event User Event {
        w202 = T13 {"Find Straight Edge_UI Command"=enum."Initialize", "Snap Simulation Mouse Down"=FALSE, "ROI Descriptor"={"Global Rectangle"=[], "Contours"=[]}, "Number of Matches Requested"=1, "Options"={"Search Direction"=0, "Edge Options"={"Edge Polarity"=0, "Kernel Size"=4, "Width"=3, "Minimum Edge Strength"=1024.0, "Interpolation Type"=enum."Zero Order", "Data Processing Method"=enum."Median"}, "Show Search Area"=FALSE, "Show Search Lines"=FALSE, "Show Edges Found"=FALSE, "Show Result"=TRUE, "Search Area Color"=5, "Search Lines Color"=3, "Edge Locations Color"=50, "Result Color"=1, "Overlay Group Name"=""}, "Line Fit Options"={"Number of Lines"=0, "Type"=enum."Best Edge Rake", "Min. Score"=0.0, "Max. Score"=25.0, "Orientation"=5.0, "Angle Range"=45.0, "Angle Tolerance"=1.0, "Step Size"=7, "Min. SNR (db)"=0.0, "Min. Points (%)"=25.0, "Hough Iterations"=5}}  # Find Straight Edge_UI Command Cluster
        n77 = event-data() -> ()  [unwired: 1 in, 1 out]
        n78 = Bundle By Name(cluster=w202, "Find Straight Edge_UI Command"=T4."Cancel" ("Barcode 1D_UI Command")) -> (w201:T13)
        n79 = Enqueue Element(queue=w200, element=w201, error in (no error)=w199) -> (error out=w198:errorcluster)  [unwired: 1 in, 2 out]
      }
      event "Cancel": Value Change {
        w206 = T13 {"Find Straight Edge_UI Command"=enum."Initialize", "Snap Simulation Mouse Down"=FALSE, "ROI Descriptor"={"Global Rectangle"=[], "Contours"=[]}, "Number of Matches Requested"=1, "Options"={"Search Direction"=0, "Edge Options"={"Edge Polarity"=0, "Kernel Size"=4, "Width"=3, "Minimum Edge Strength"=1024.0, "Interpolation Type"=enum."Zero Order", "Data Processing Method"=enum."Median"}, "Show Search Area"=FALSE, "Show Search Lines"=FALSE, "Show Edges Found"=FALSE, "Show Result"=TRUE, "Search Area Color"=5, "Search Lines Color"=3, "Edge Locations Color"=50, "Result Color"=1, "Overlay Group Name"=""}, "Line Fit Options"={"Number of Lines"=0, "Type"=enum."Best Edge Rake", "Min. Score"=0.0, "Max. Score"=25.0, "Orientation"=5.0, "Angle Range"=45.0, "Angle Tolerance"=1.0, "Step Size"=7, "Min. SNR (db)"=0.0, "Min. Points (%)"=25.0, "Hough Iterations"=5}}  # Find Straight Edge_UI Command Cluster
        n80 = event-data() -> ()  [unwired: 1 in, 1 out]
        n81 = Bundle By Name(cluster=w206, "Find Straight Edge_UI Command"=T4."Cancel" ("Barcode 1D_UI Command")) -> (w205:T13)
        n82 = Enqueue Element(queue=w211, element=w205, error in (no error)=w210) -> (error out=w208:errorcluster)  [unwired: 1 in, 2 out]
      }
      event "Snap?": Value Change {
        w213 = T13 {"Find Straight Edge_UI Command"=enum."Initialize", "Snap Simulation Mouse Down"=FALSE, "ROI Descriptor"={"Global Rectangle"=[], "Contours"=[]}, "Number of Matches Requested"=1, "Options"={"Search Direction"=0, "Edge Options"={"Edge Polarity"=0, "Kernel Size"=4, "Width"=3, "Minimum Edge Strength"=1024.0, "Interpolation Type"=enum."Zero Order", "Data Processing Method"=enum."Median"}, "Show Search Area"=FALSE, "Show Search Lines"=FALSE, "Show Edges Found"=FALSE, "Show Result"=TRUE, "Search Area Color"=5, "Search Lines Color"=3, "Edge Locations Color"=50, "Result Color"=1, "Overlay Group Name"=""}, "Line Fit Options"={"Number of Lines"=0, "Type"=enum."Best Edge Rake", "Min. Score"=0.0, "Max. Score"=25.0, "Orientation"=5.0, "Angle Range"=45.0, "Angle Tolerance"=1.0, "Step Size"=7, "Min. SNR (db)"=0.0, "Min. Points (%)"=25.0, "Hough Iterations"=5}}  # Find Straight Edge_UI Command Cluster
        n83 = event-data() -> ("NewVal"=w212:bool)  [unwired: 1 in, 1 out]
        n84 = case shown="True" w212 {
          tunnel: w216 -> [_ w226]
          tunnel: w215 -> [w217 w225]
          tunnel: w213 -> [_ w223]
          tunnel: [w217 w222] -> w214
          frame False {
          }
          frame True {
            n85 = Bundle By Name(cluster=w223, "Find Straight Edge_UI Command"=T4."Initialize" ("Barcode 1D_UI Command"), "Snap Simulation Mouse Down"=TRUE) -> (w221:T13)
            n86 = Enqueue Element(queue=w226, element=w221, error in (no error)=w225) -> (queue out=w219:refnum<queue>, error out=w218:errorcluster)  [unwired: 1 in, 1 out]
            n87 = disable-structure shown="Disabled" {
              disable-tunnel: w223 -> [w236 _]
              disable-tunnel: [w235 _] -> w222
              disable-tunnel: w219 -> [w234 _]
              disable-tunnel: w218 -> [w233 _]
              frame Disabled {
                n88 = local read "ROI"() -> (w227:T1)
                n89 = local read item#-1() -> (w229)
                n90 = local read item#-1() -> (w230)
                n91 = local read item#-1() -> (w231)
                n92 = Bundle By Name(cluster=w236, "Clamp MAX_UI Command"=T4."Run Algorithm" ("Barcode 1D_UI Command"), "Overlay Settings"=w231, "Curve Extraction Settings"=w230, "Clamp Settings"=w229, "ROI"=w227) -> (w228:T13)
                n93 = Enqueue Element(queue=w234, element=w228, error in (no error)=w233) -> (error out=w235:errorcluster)  [unwired: 1 in, 2 out]
              }
              frame Enabled {
              }
            }
          }
        }
      }
    }
  }
  n94 = Unregister For Events(event registration refnum=w5) -> ()  [unwired: 1 in, 1 out]
  n95 = Destroy User Event(user event=w3, error in=w2) -> (error out=w1:errorcluster)
  n96 = Merge Errors(w15, w1) -> (→"error out":errorcluster)
